vi "CompositeProperties.vi"(0 "Image Reference":refnum<vi>, 1 "Ramp Reference":refnum<vi>, 2 "Pixel Size":i32, 3 "Max Lifetime (s)":dbl=4e-09, 4 "Min Lifetime (s)":dbl=1e-09, 5 "error in (no error)":errorcluster) -> (19 "error out":errorcluster)   [LabVIEW 2015]
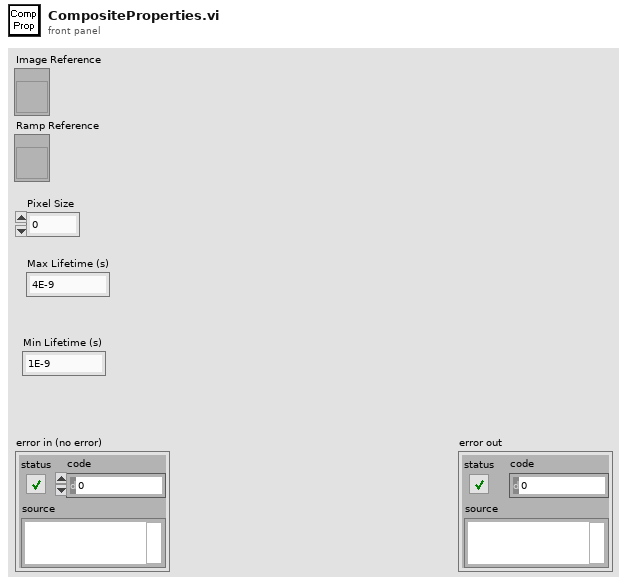
[diagram p1: front panel]
types:
  T1 = typedef "LVBoundsTypeDef.ctl" = cluster{"Width":u32, "Height":u32}
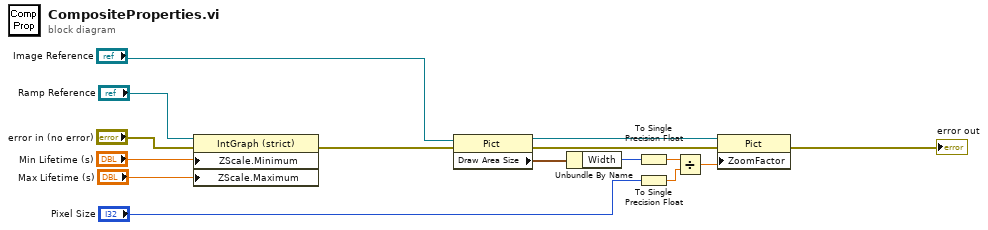
[diagram p0: block diagram]
diagram:
  n1 = property class="IntGraph (strict)"(reference="Ramp Reference", error in="error in (no error)", "ZScale.Minimum"="Min Lifetime (s)", "ZScale.Maximum"="Max Lifetime (s)") -> (error out=w8:errorcluster)  [unwired: 1 out]
  n2 = property class="Pict"(reference="Image Reference", error in=w8) -> (reference out=w9:refnum<vi>, error out=w10:errorcluster, "Draw Area Size"=w12:T1)
  n3 = Unbundle By Name(w12) -> ("Width"=w13:u32)
  n4 = To Single Precision Float(number=w13) -> (single precision float=w15:sgl)
  n5 = To Single Precision Float(number="Pixel Size") -> (single precision float=w14:sgl)
  n6 = Divide(x=w15, y=w14) -> (x/y=w11:sgl)
  n7 = property class="Pict"(reference=w9, error in=w10, "ZoomFactor"=w11) -> (error out=→"error out":errorcluster)  [unwired: 1 out]
